vi "B29xx_auto_ohms.vi"(6 "Resistance Auto Range (T: Enable)":bool=TRUE, 7 "Enable Remote Sensing (4-wire)":bool=TRUE, 11 "SMU VISA name":refnum<visa-resource-name>="GPIB1::29::INSTR") -> (2 "Measured Resistance (Ohms)":dbl format="%#_6p")   [LabVIEW 2020]
uses:
  <instrlib>/Agilent B2900 Series/Public/Configure/Measurement/Configure Measurement (Resistance).vi
  <instrlib>/Agilent B2900 Series/Agilent B2900 Series.lvlib
panel:
  in  "Resistance Range Lower Limit (2 Ohm)":dbl=2.0 format="%#_6p"
  in  "Resistance Range Upper Limit (2E+8 Ohm)":dbl=200000000.0 format="%#_6p"
  in  "Resistance NPLC (0.1)":dbl=0.1
  in  "Resistance Range (2 Ohm)":dbl=2.0
  in  "Error In":errorcluster
  # "Keysight B29xx - Auto Resistance Measurement  (Remote Sensing)"
  # "If Auto Range Disabled use Manual Range.."
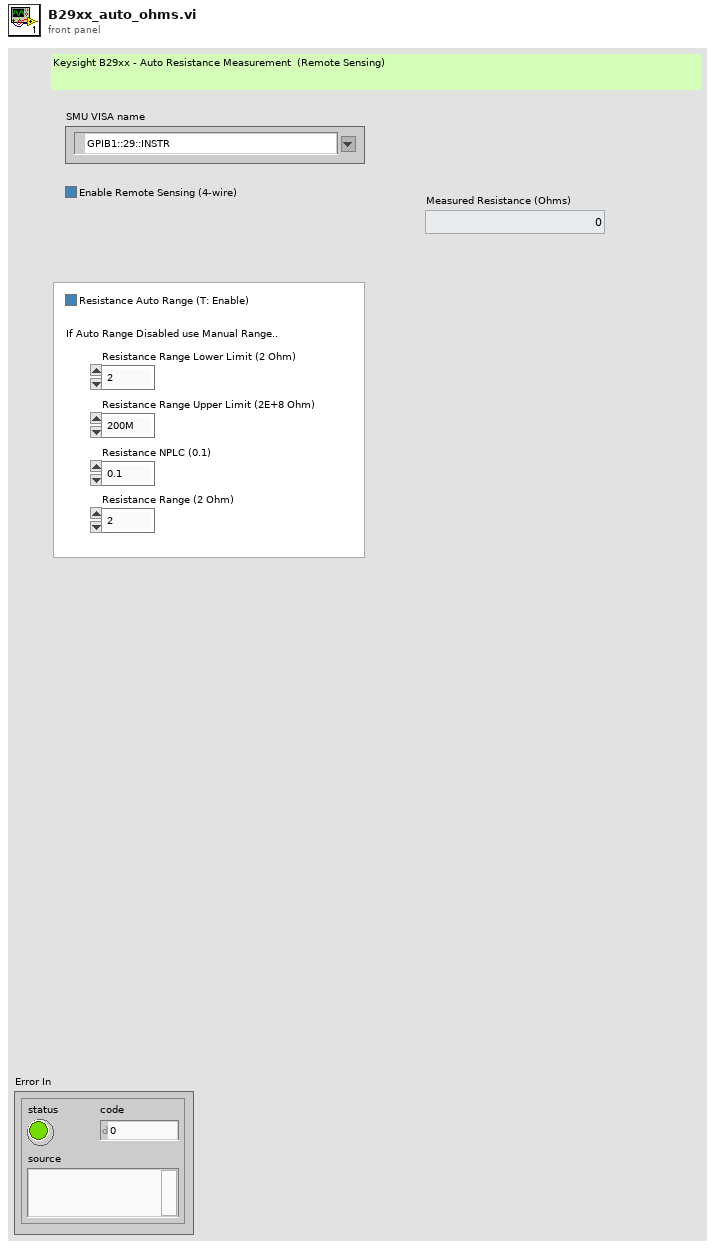
[diagram p1: front panel]
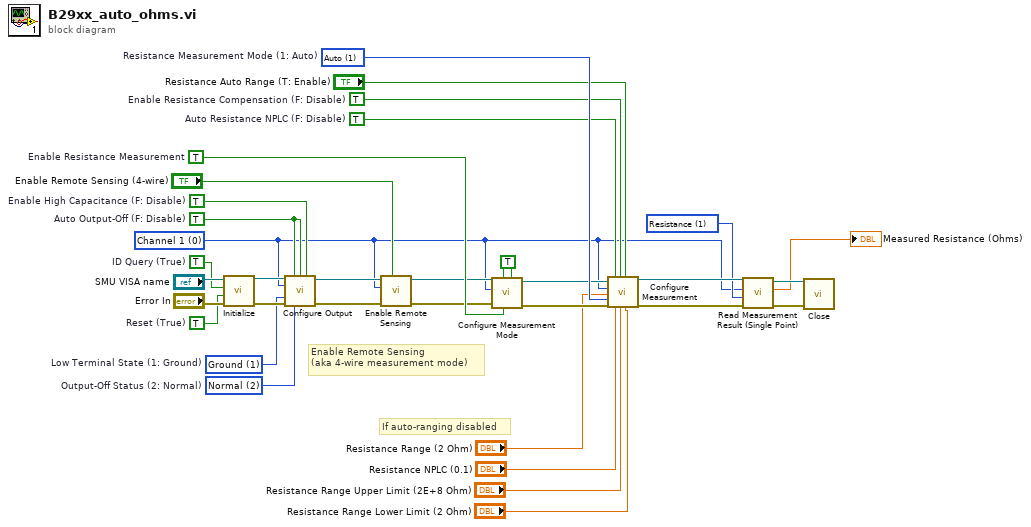
[diagram p0: block diagram]
diagram:
  w5 = 1 items=["Current", "Resistance", "Source Output Setting", "Status", "Time", "Voltage"] ("Data Mode (5: Voltage)")
  w16 = TRUE ("Enable Voltage Measurement (T: Enable)")
  w17 = TRUE  # Enable Resistance Measurement
  w19 = TRUE  # Enable Resistance Compensation (F: Disable)
  w20 = TRUE  # Auto Resistance NPLC (F: Disable)
  w21 = TRUE  # Enable High Capacitance (F: Disable)
  w22 = 1 items=["Manual", "Auto"]  # Resistance Measurement Mode (1: Auto)
  w23 = 2 items=["Zero", "HIZ", "Normal"]  # Output-Off Status (2: Normal)
  w24 = 1 items=["Float", "Ground"]  # Low Terminal State (1: Ground)
  w25 = TRUE  # Auto Output-Off (F: Disable)
  w4 = 0 items=["Channel 1", "Channel 2"] ("Channel (0: Channel 1)")
  w28 = TRUE  # ID Query (True)
  w29 = TRUE  # Reset (True)
  # "If auto-ranging disabled"
  # "Enable Remote Sensing\n(aka 4-wire measurement mode)"
  n1 = call <instrlib>:"Initialize.vi"("error in (no error)"="Error In", "Reset (True)"=w29, "ID Query (True)"=w28, "VISA resource name"="SMU VISA name") -> ("error out"=w27:errorcluster, "VISA resource name out"=w26:refnum<visa-resource-name>)  [unwired: 6 in]
  n2 = call <instrlib>:"Configure Output.vi"("VISA resource name"=w26, "Auto Output-Off (F: Disable)"=w25, "Auto Output-On (T: Enable)"=w25, "Enable High Capacitance (F: Disable)"=w21, "Channel (0: Channel 1)"=w4, "Low Terminal State (1: Ground)"=w24, "error in (no error)"=w27, "Output-Off Status (2: Normal)"=w23) -> ("VISA resource name out"=w32:refnum<visa-resource-name>, "error out"=w33:errorcluster)  [unwired: 6 in]
  n3 = call <instrlib>:"Enable Remote Sensing.vi"("Enable Remote Sensing (F: Disable)"="Enable Remote Sensing (4-wire)", "error in (no error)"=w33, "Channel (0: Channel 1)"=w4, "VISA resource name"=w32) -> ("error out"=w7:errorcluster, "VISA resource name out"=w6:refnum<visa-resource-name>)  [unwired: 6 in]
  n4 = call <instrlib>:"Configure Measurement Mode.vi"("Enable Current Measurement (T: Enable)"=w16, "Enable Resistance Measurement (F: Disable)"=w17, "Enable Voltage Measurement (T: Enable)"=w16, "error in (no error)"=w7, "Channel (0: Channel 1)"=w4, "VISA resource name"=w6) -> ("error out"=w15:errorcluster, "VISA resource name out"=w14:refnum<visa-resource-name>)  [unwired: 4 in]
  n5 = call-poly <instrlib>:"Configure Measurement.vi"("VISA resource name"=w14, "Channel (0: Channel 1)"=w4, "Resistance Range (2 Ohm)"="Resistance Range (2 Ohm)", "Resistance Measurement Mode (1: Auto)"=w22, "error in (no error)"=w15, "Auto Resistance NPLC (F: Disable)"=w20, "Resistance NPLC (0.1)"="Resistance NPLC (0.1)", "Enable Resistance Compensation (F: Disable)"=w19, "Resistance Range Upper Limit (2E+8 Ohm)"="Resistance Range Upper Limit (2E+8 Ohm)", "Resistance Auto Range (T: Enable)"="Resistance Auto Range (T: Enable)", "Resistance Range Lower Limit (2 Ohm)"="Resistance Range Lower Limit (2 Ohm)") -> ("VISA resource name out"=w12:refnum<visa-resource-name>, "error out"=w13:errorcluster)  [unwired: 7 in]
  n6 = call <instrlib>:"Read Measurement Result (Single Point).vi"("error in (no error)"=w13, "Data Mode (5: Voltage)"=w5, "Channel (0: Channel 1)"=w4, "VISA resource name"=w12) -> ("error out"=w2:errorcluster, "Measurement Result"=→"Measured Resistance (Ohms)":dbl, "VISA resource name out"=w3:refnum<visa-resource-name>)  [unwired: 5 in]
  n7 = call <instrlib>:"Close.vi"("error in (no error)"=w2, "VISA resource name"=w3) -> ()  [unwired: 9 in, 1 out]
